vi "New Message Queue.vi"(8 "error in (no error)":errorcluster, 11 "ModuleName In":T1=enum."Controller") -> (0 "error out":errorcluster, 3 "Msg queue out":refnum<queue>)   [LabVIEW 2021, in "Architecture.lvlib"]
doc: "This method creates a queue based on a module name and a tick count (in case we can have any module cloned)."
uses:
  Architecture.lvlib
  Typedefs/Enum_Module_Name.ctl
  Typedefs/Message.ctl
  Modules/Configuration/Configuration.lvlib
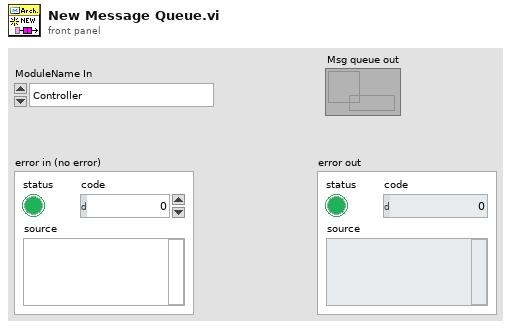
[diagram p1: front panel]
types:
  T1 = typedef "Configuration.lvlib/Enum_Module_Name.ctl" = enum16{"Configuration", "Error_Handler", "Log", "Database", "Controller", "UI Module", "Sound Manager"}
  T2 = typedef "Architecture.lvlib/Message.ctl" = cluster{"Message":string, "Data":variant, "syn":bool}
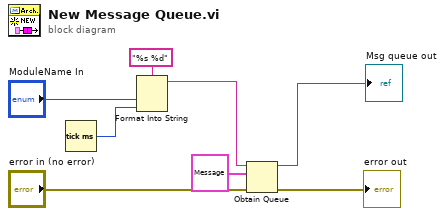
[diagram p0: block diagram]
diagram:
  n1 = Tick Count (ms)() -> (millisecond timer value=w6:u32)
  n2 = Format Into String(format string="%s %d", "ModuleName In", w6) -> (resulting string=w7:string)  [unwired: 2 in, 1 out]
  n3 = Obtain Queue(name (unnamed)=w7, element data type=T2 {"Message"="", "Data"=variant, "syn"=FALSE} ("Message"), error in (no error)="error in (no error)") -> (queue out=→"Msg queue out":refnum<queue>, error out=→"error out":errorcluster)  [unwired: 2 in, 1 out]
